vi "Generate SineWave.vi"(1 "GenSine":bool) -> (0 "Sine Point":sgl)   [LabVIEW 2020]
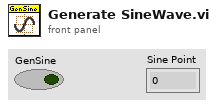
[diagram p1: front panel]
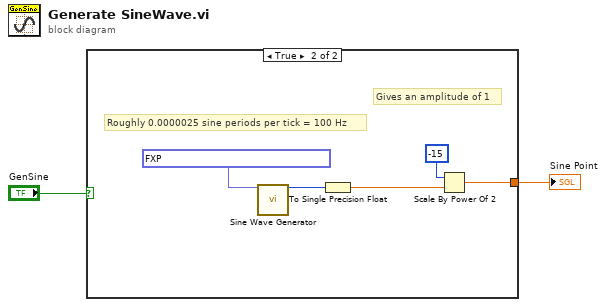
[diagram p0: block diagram]
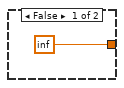
[diagram p2: hidden frame]
diagram:
  n1 = case shown="True" "GenSine" {
    tunnel: [sgl inf w8] -> w2
    frame False {
    }
    frame True {
      # "Gives an amplitude of 1"
      # "Roughly 0.0000025 sine periods per tick = 100 Hz"
      n2 = call "Sine Wave Generator"("frequency (periods/tick)"=fxp<+,32,0> 2.499902620911598e-06) -> ("sine out"=w5:i16)  [unwired: 14 in]
      n3 = To Single Precision Float(number=w5) -> (single precision float=w6:sgl)
      n4 = Scale By Power Of 2(n=i16 -15, x=w6) -> (x*2^n=w8:sgl)
    }
  }
  "Sine Point" <- w2
